vi "SubtractRings.vi"(2 "delay pts":i32[][](array[numeric]), 3 "h(r,t) ring inner":dbl[][](array[numeric]) format="%.2f", 4 "h(r,t) ring outer":dbl[][](array[numeric]) format="%.2f") -> (0 "h(r,t) annulus":dbl[][](array[numeric]) format="%.2f", 1 "delay pts out":i32[](array[numeric]))   [LabVIEW 2022 SP3]
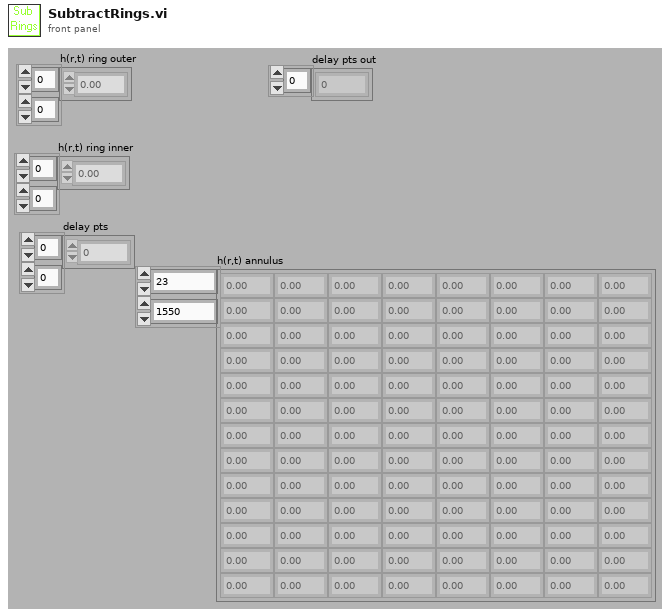
[diagram p1: front panel]
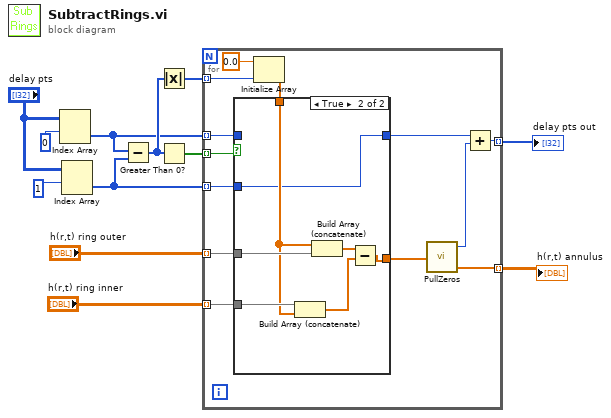
[diagram p0: block diagram]
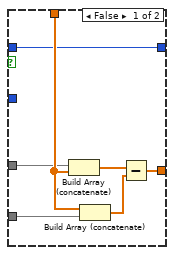
[diagram p2: hidden frame]
diagram:
  n1 = Index Array(array="delay pts", index (row)=0) -> (element=w3:i32[])  [unwired: 1 in]
  n2 = Index Array(array="delay pts", index (row)=1) -> (element=w4:i32[])  [unwired: 1 in]
  n3 = Subtract(x=w3, y=w4) -> (x-y=w8:i32[])
  n4 = Absolute Value(x=w8) -> (abs(x)=w7:i32[])
  n5 = Greater Than 0?(x=w8) -> (x > 0?=w9:bool[])
  n6 = for {
    tunnel: "h(r,t) ring outer" -> [w19] mode=indexing
    tunnel: "h(r,t) ring inner" -> [w18] mode=indexing
    tunnel: [w13] -> w1 mode=indexing
    tunnel: w9 -> [w23] mode=indexing
    tunnel: w7 -> [w22] mode=indexing
    tunnel: w4 -> [w21] mode=indexing
    tunnel: w3 -> [w20] mode=indexing
    tunnel: [w14] -> w2 mode=indexing
    n7 = Initialize Array(0.0, w22) -> (w24:dbl[])
    n8 = case shown="True" w23 {
      tunnel: w19 -> [w27 w39]
      tunnel: w18 -> [w26 w37]
      tunnel: w24 -> [w31 w36]
      tunnel: [w32 w38] -> w17
      tunnel: w21 -> [_ w33]
      tunnel: w20 -> [w28 _]
      tunnel: [w28 w33] -> w15
      frame False {
        n9 = Build Array (concatenate)(w27, w31) -> (w30:dbl[])
        n10 = Build Array (concatenate)(w31, w26) -> (w29:dbl[])
        n11 = Subtract(x=w30, y=w29) -> (x-y=w32:dbl[])
      }
      frame True {
        n12 = Build Array (concatenate)(w37, w36) -> (w34:dbl[])
        n13 = Build Array (concatenate)(w36, w39) -> (w35:dbl[])
        n14 = Subtract(x=w35, y=w34) -> (x-y=w38:dbl[])
      }
    }
    n15 = call "PullZeros.vi"("input"=w17) -> ("output"=w13:dbl[], "pre-zeros"=w16:i32)  [unwired: 3 out]
    n16 = Add(x=w15, y=w16) -> (x+y=w14:i32)
  }
  "delay pts out" <- w2
  "h(r,t) annulus" <- w1
